vi "Send and Receive.vi"(8 "error in (no error)":errorcluster, 10 "Command":string, 11 "EPU452 in":refnum<class "EPU452.lvclass">) -> (0 "error out":errorcluster, 2 "Response":string, 3 "EPU452 out":refnum<class "EPU452.lvclass">)   [LabVIEW 2018, in "EPU452.lvclass"]
uses:
  EPU452.lvclass
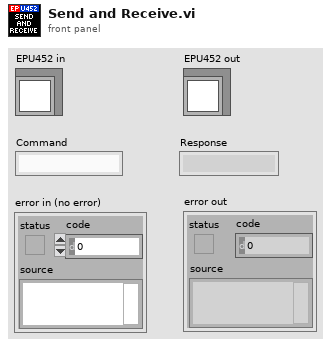
[diagram p1: front panel]
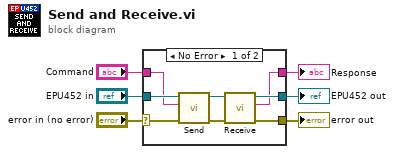
[diagram p0: block diagram]
diagram:
  n1 = case shown="No Error" "error in (no error)" {
    selector: "error in (no error)" -> [w9 w16]
    tunnel: [w11 w16] -> w5
    tunnel: [w12 w15] -> w3
    tunnel: "EPU452 in" -> [w8 w15]
    tunnel: "Command" -> [w7 _]
    tunnel: [w10 _] -> w1
    frame No Error {
      n2 = call "Send.vi"("error in (no error)"=w9, "Command"=w7, "EPU452 in"=w8) -> ("error out"=w13:errorcluster, "EPU452 out"=w14:refnum<class "EPU452.lvclass">)  [unwired: 7 in]
      n3 = call "Receive.vi"("error in (no error)"=w13, "EPU452 in"=w14) -> ("error out"=w11:errorcluster, "Response"=w10:string, "EPU452 out"=w12:refnum<class "EPU452.lvclass">)  [unwired: 7 in]
    }
    frame Error {
    }
  }
  "error out" <- w5
  "EPU452 out" <- w3
  "Response" <- w1
